vi "Log Run.vi"(8 "error in (no error)":errorcluster, 11 "CIFCorePlugin in":refnum<class "CIFCorePlugin.lvclass">) -> (0 "error out":errorcluster, 3 "CIFCorePlugin out":refnum<class "CIFCorePlugin.lvclass">)   [LabVIEW 2021, in "CIFCorePlugin.lvclass"]
uses:
  CIFCorePlugin.lvclass
  CIFCorePlugin.lvclass/CIFCorePlugin.ctl
  CIFUtilities/CIFLogs/Typedef/Plugin State Commands.ctl
  CIFUtilities/CIFLogs/CIFLogs.lvlib
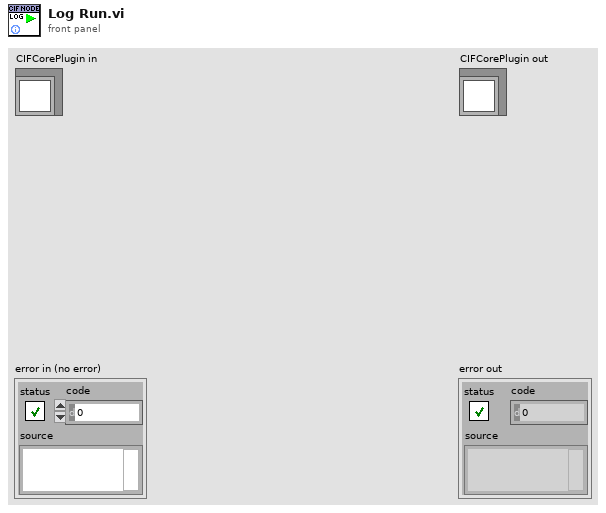
[diagram p1: front panel]
types:
  T1 = typedef "CIFLogs.lvlib/Plugin State Commands.ctl" = enum16{"Create", "Configure", "Run", "Pause", "Destroy"}
  T2 = typedef "CIFCorePlugin.lvclass/Energized States.ctl" = enum16{"Listen", "Prepare", "Execute", "Housekeep", "Cleanup", "Destroy"}
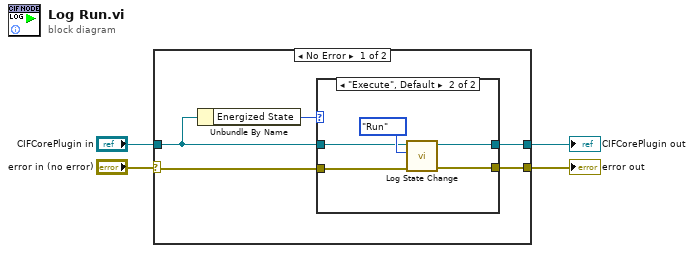
[diagram p0: block diagram]
diagram:
  n1 = case shown="No Error" "error in (no error)" {
    selector: "error in (no error)" -> [w8 w18]
    tunnel: [w7 w18] -> w3
    tunnel: [w9 w17] -> w1
    tunnel: "CIFCorePlugin in" -> [w6 w17]
    frame No Error {
      n2 = Unbundle By Name(w6) -> ("Energized State"=w5:T2)
      n3 = case shown="\"Execute\", Default" w5 {
        tunnel: [w11 w15] -> w9
        tunnel: w8 -> [w10 w14]
        tunnel: [w10 w13] -> w7
        tunnel: w6 -> [w11 w12]
        frame "Destroy" {
        }
        frame "Execute", Default {
          n4 = call "Log State Change.vi"("error in (no error)"=w14, "Command"=Plugin_State_Commands."Run", "CIFCorePlugin in"=w12) -> ("error out"=w13:errorcluster, "CIFCorePlugin out"=w15:refnum<class "CIFCorePlugin.lvclass">)  [unwired: 7 in]
        }
      }
    }
    frame Error {
    }
  }
  "error out" <- w3
  "CIFCorePlugin out" <- w1
